vi "WFS Get Mla Data.vi"(0 "instrument handle":refnum<visa-resource-name>, 7 "MLA Index":i32 format="%.0g", 11 "error in (no error)":errorcluster {"code" format="%.0x"}) -> (2 "Grd Corr 0":dbl, 3 "Spot Offset Y":dbl, 4 "instrument handle out":refnum<visa-resource-name>, 6 "MLA Name":string, 8 "Cam Pitch µm":dbl, 10 "Lenslet Pitch µm":dbl, 12 "Grd Corr 45":dbl, 13 "Lenslet f µm":dbl, 14 "Spot Offset X":dbl, 15 "error out":errorcluster {"code" format="%.0x"})   [LabVIEW 2020]
doc: "This VI returns calibration data of the desired Microlens Array index. The number of calibrated lenslet arrays can be derived by VI GetMlaCals.\n\nNote: The calibration data are not automatically set active."
uses:
  WFS_32.dll
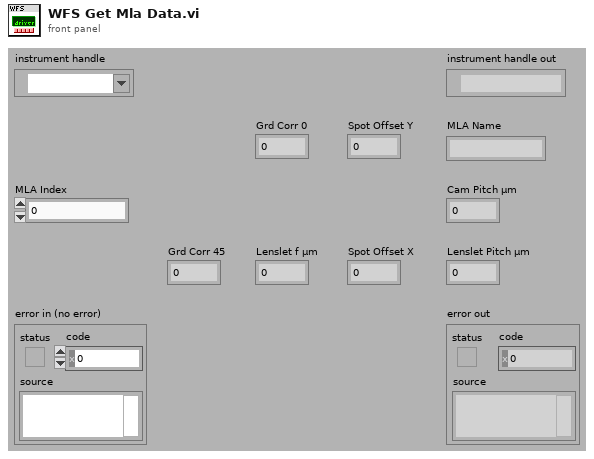
[diagram p1: front panel]
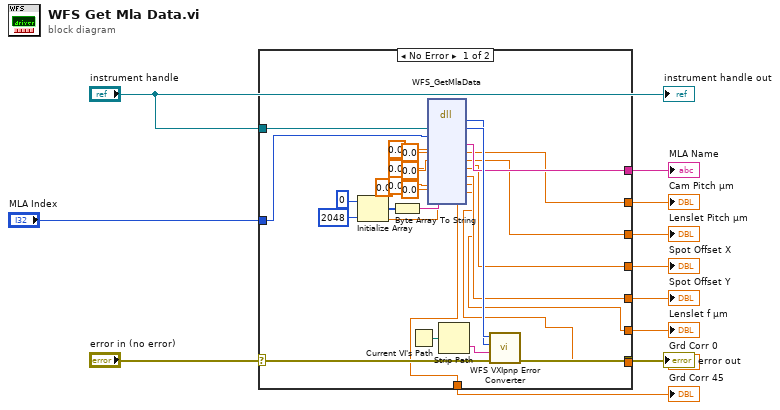
[diagram p0: block diagram]
diagram:
  n1 = case shown="No Error" "error in (no error)" {
    selector: "error in (no error)" -> [w34 w40]
    tunnel: [w33 w40] -> w12
    tunnel: "instrument handle" -> [w38 _]
    tunnel: "MLA Index" -> [w32 _]
    tunnel: [w27 _] -> w8
    tunnel: [w25 _] -> w7
    tunnel: [w23 _] -> w6
    tunnel: [w21 _] -> w5
    tunnel: [w19 _] -> w4
    tunnel: [w17 _] -> w3
    tunnel: [w15 _] -> w2
    tunnel: [w13 _] -> w1
    frame No Error {
      n2 = Initialize Array(u8 0 ("element"), 2048 ("dimension size")) -> (w30:u8[])
      n3 = Byte Array To String(unsigned byte array=w30) -> (string=w31:string)
      n4 = Current VI's Path() -> (path=w39:path)
      n5 = dll-call lib="WFS_*.*" fn="WFS_GetMlaData"("Instrument Handle"=w38, "MLA Index"=w32, "MLA Name"=w31, "Cam Pitch µm"=0.0, "Lenslet Pitch µm"=0.0, "Spot Offset X"=0.0, "Spot Offset Y"=0.0, "Lenslet f µm"=0.0, "Grd Corr 0"=0.0, "Grd Corr 45"=0.0) -> (w36:i32, "Instrument Handle"=w37:u32, "MLA Name"=w27:string, "Cam Pitch µm"=w25:dbl, "Lenslet Pitch µm"=w23:dbl, "Spot Offset X"=w21:dbl, "Spot Offset Y"=w19:dbl, "Lenslet f µm"=w17:dbl, "Grd Corr 0"=w15:dbl, "Grd Corr 45"=w13:dbl)  [unwired: 4 in, 2 out]
      n6 = Strip Path(path=w39) -> (name=w35:string)  [unwired: 1 out]
      n7 = call "WFS VXIpnp Error Converter.vi"("error in (no error)"=w34, "Name Of VI (\"\")"=w35, "CVI Error Code (0)"=w36, "instrument handle"=w37) -> ("error out"=w33:errorcluster)  [unwired: 6 in, 1 out]
    }
    frame Error {
    }
  }
  "error out" <- w12
  "MLA Name" <- w8
  "Cam Pitch µm" <- w7
  "Lenslet Pitch µm" <- w6
  "Spot Offset X" <- w5
  "Spot Offset Y" <- w4
  "Lenslet f µm" <- w3
  "Grd Corr 0" <- w2
  "Grd Corr 45" <- w1
  "instrument handle out" <- "instrument handle"
